vi "init_station_keeping.vi"(6 "Buoy SE":T1 {"North" format="%#_10f"; "East" format="%#_8f"}, 7 "Buoy NE":T1 {"North" format="%#_10f"; "East" format="%#_8f"}, 8 "Buoy SW":T1 {"North" format="%#_10f"; "East" format="%#_8f"}, 11 "Buoy NW":T1 {"North" format="%#_10f"; "East" format="%#_8f"}) -> (3 "Mission out":refnum<class "Mission.lvclass">)   [LabVIEW 2011, in "Mission.lvclass"]
uses:
  Mission.lvclass
  2 Typedefs/UTM Location.ctl
  Mission.lvclass/Mission.ctl
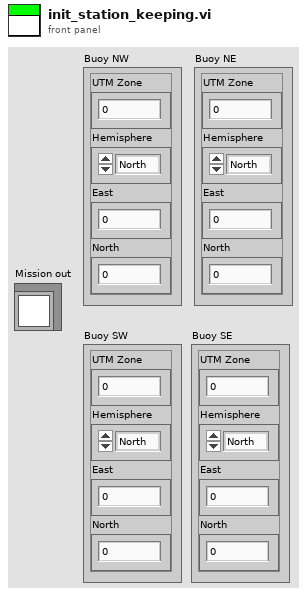
[diagram p1: front panel]
types:
  T1 = typedef "UTM Location.ctl" = cluster{"UTM Zone":dbl, "Hemisphere":enum16{"North", "South"}, "East":dbl, "North":dbl}
  T2 = enum16{"Round Buoy", "Drive", "Pass Buoys", "Station Keeping"}
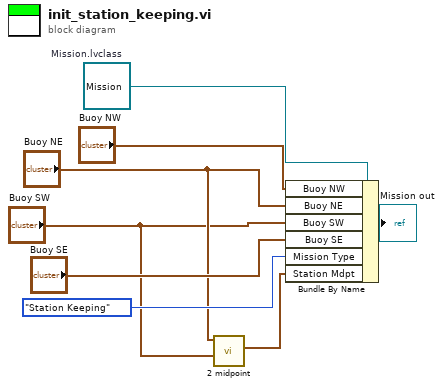
[diagram p0: block diagram]
diagram:
  w8 = refnum<class "Mission.lvclass"> refnum  # Mission.lvclass
  n1 = call "2 midpoint.vi"("UTM 2"="Buoy SW", "UTM 1"="Buoy NE") -> ("Midpoint"=w3:T1)  [unwired: 9 in]
  n2 = Bundle By Name(cluster=w8, "Buoy NW"="Buoy NW", "Buoy NE"="Buoy NE", "Buoy SW"="Buoy SW", "Buoy SE"="Buoy SE", "Mission Type"=T2."Station Keeping", "Station Mdpt"=w3) -> (→"Mission out":refnum<class "Mission.lvclass">)
